vi "connect.vi"(8 "error in (no error)":errorcluster, 11 "comic_class in":refnum<class "comic_class.lvclass">) -> (0 "error out":errorcluster, 3 "comic_class out":refnum<class "comic_class.lvclass">)   [LabVIEW 2024, in "comic_class.lvclass"]
uses:
  comic_class.lvclass
  comic_class.lvclass/comic_class.ctl
  <vilib>/httpClient/POSTBuffer.vi
  <vilib>/httpClient/LabVIEWHTTPClient.lvlib
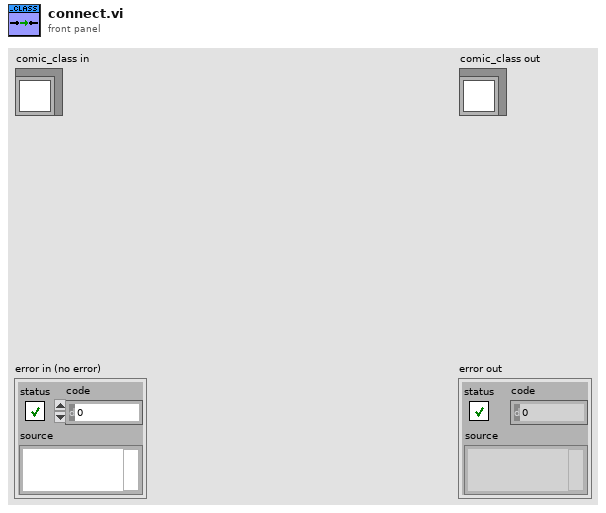
[diagram p1: front panel]
types:
  T1 = typedef "LabVIEWHTTPClient.lvlib/ClientHandle.ctl" = refnum<k1>
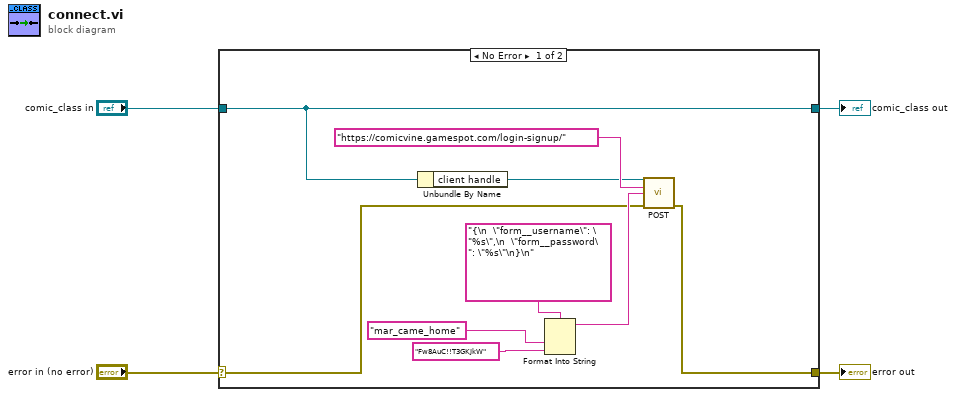
[diagram p0: block diagram]
diagram:
  n1 = case shown="No Error" "error in (no error)" {
    selector: "error in (no error)" -> [w6 w15]
    tunnel: [w5 w15] -> w3
    tunnel: [w7 w14] -> w1
    tunnel: "comic_class in" -> [w7 w14]
    frame No Error {
      n2 = Unbundle By Name(w7) -> ("client handle"=w8:T1)
      n3 = Format Into String(format string="{\n  \"form__username\": \"%s\",\n  \"form__password\": \"%s\"\n}\n", "mar_came_home", "Fw8AuC!!T3GKJkW") -> (resulting string=w10:string)  [unwired: 2 in, 1 out]
      n4 = call-poly <vilib>:"POST.vi"("client handle"=w8, "url"="https://comicvine.gamespot.com/login-signup/", "buffer"=w10, "error in (no error)"=w6) -> ("error out"=w5:errorcluster)  [unwired: 8 in, 3 out]
    }
    frame Error {
    }
  }
  "error out" <- w3
  "comic_class out" <- w1
